vi "macro_LinearSystemLoop_Elevator_Execute.vi"() -> ()   [LabVIEW 2019, in "Trajectory_Library.lvlib"]
uses:
  Trajectory_Library.lvlib
  Enum/DCMOTOR_TYPES_ENUM.ctl
panel:
  in  "MeasHeight PV M":dbl
  in  "Height SP M":dbl
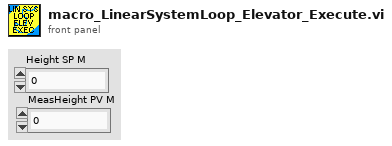
[diagram p1: front panel]
types:
  T1 = typedef "Trajectory_Library.lvlib/DCMOTOR_TYPES_ENUM.ctl" = enum16{"CIM", "AndyMark 9015", "Andy Mark RS 775 125", "Bag", "BaneBots RS 550", "BaneBots RS 775", "Falcon 500", "Mini CIM", "NEO", "NEO 550", "Romi BuiltIn", "Vex 775 Pro", "Snow Blower AM 2235A", "Bosch Seat AM 3493"}
  T2 = typedef "Trajectory_Library.lvlib/LINEAR_SYSTEM_ID_ELEVATOR_MODEL.CTL" = cluster{"DCMOTOR_TYPES":T1, "Num Motors":i32, "WinchRadias_Meters":dbl, "mass_Kg":dbl, "Gearing":dbl}
  T3 = typedef "Trajectory_Library.lvlib/LINEAR_SYSTEM_LOOP_ELEVATOR_CTRL_PARAMS.CTL" = cluster{"Pos Model Std Dev M":dbl, "Vel Model Std Dev M/S":dbl, "Pos Meas Std Dev M":dbl, "Pos Ctrl Tol M":dbl, "Vel Ctrl Tol M/S":dbl, "Max Ctrl Out V":dbl}
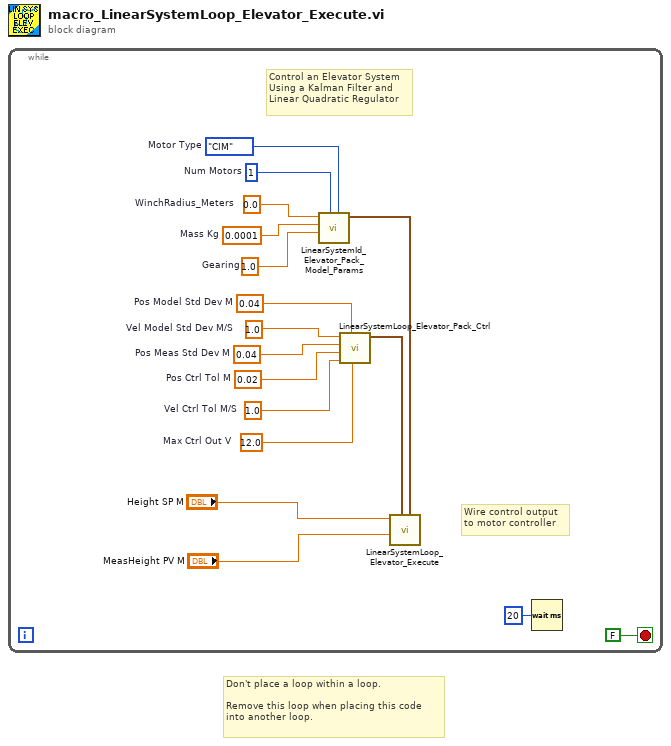
[diagram p0: block diagram]
diagram:
  # "Don't place a loop within a loop.\n \nRemove this loop when placing this code\ninto another loop."
  n1 = while {
    stop <- FALSE stop-if-true
    w1 = 1.0  # Vel Model Std Dev M/S
    w2 = 0.04  # Pos Meas Std Dev M
    w3 = 0.02  # Pos Ctrl Tol M
    w4 = 1.0  # Vel Ctrl Tol M/S
    w5 = 0.04  # Pos Model Std Dev M
    w6 = 12.0  # Max Ctrl Out V
    w11 = 0.0  # WinchRadius_Meters
    w14 = 1.0  # Gearing
    w15 = 0.0001  # Mass Kg
    w16 = 1  # Num Motors
    w17 = DCMOTOR_TYPES_ENUM."CIM"  # Motor Type
    # "Wire control output\nto motor controller"
    # "Control an Elevator System\nUsing a Kalman Filter and \nLinear Quadratic Regulator"
    n2 = call "LinearSystemId_Elevator_Pack_Model_Params.vi"("DCMOTOR_TYPES"=w17, "Num Motors"=w16, "Gearing"=w14, "mass_Kg"=w15, "WinchRadius_Meters"=w11) -> ("Elevator_Model _Params"=w10:T2)  [unwired: 6 in]
    n3 = call "LinearSystemLoop_Elevator_Pack_Ctrl.vi"("Max Ctrl Out V"=w6, "Pos Model Std Dev M"=w5, "Vel Ctrl Tol M/S"=w4, "Pos Ctrl Tol M"=w3, "Pos Meas Std Dev M"=w2, "Vel Model Std Dev M/S"=w1) -> ("LinearSystemLoop_Elevator_Ctrl_Params"=w9:T3)  [unwired: 5 in]
    n4 = call "LinearSystemLoop_Elevator_Execute.vi"("ElevatorSim_Model _Params"=w10, "LinearSystem_Elevator_Ctrl_Params"=w9, "RawHeight PV"="MeasHeight PV M", "Height SP"="Height SP M") -> ()  [unwired: 4 in, 4 out]
    n5 = Wait (ms)(milliseconds to wait=u32 20) -> ()  [unwired: 1 out]
  }
